vi "RSA306 FFT sweeper2.vi"(0 "Q Array":sgl[](array[numeric]), 1 "2nd Cursor X":dbl, 2 "1st Cursor X":dbl, 3 "Time Array":dbl[](array[numeric]), 5 "1toN Array":i32[](array[numeric]), 7 "I Array":sgl[](array[numeric]), 9 "time step(sec)":dbl, 12 "Freq Center":dbl, 13 "Use windowing":bool, 14 "beta":dbl format="%0.2f") -> (4 "# of Pts Between cursors":dbl, 6 "I & Q  partial":cluster{dbl[], sgl[]}[](graph), 8 "Length out":i32, 10 "FFT^2 from partial":cluster{dbl[], dbl[]}, 15 "FreqStep":dbl)   [LabVIEW 2016]
uses:
  <vilib>/Analysis/4window.llb/Kaiser-Bessel Window (CDB).vi
  <vilib>/Analysis/2dsp.llb/Complex FFT.vi
  <vilib>/Analysis/NI_AALPro.lvlib
panel:
  out "FFT^2  partial":cluster{dbl[], dbl[]}(graph)
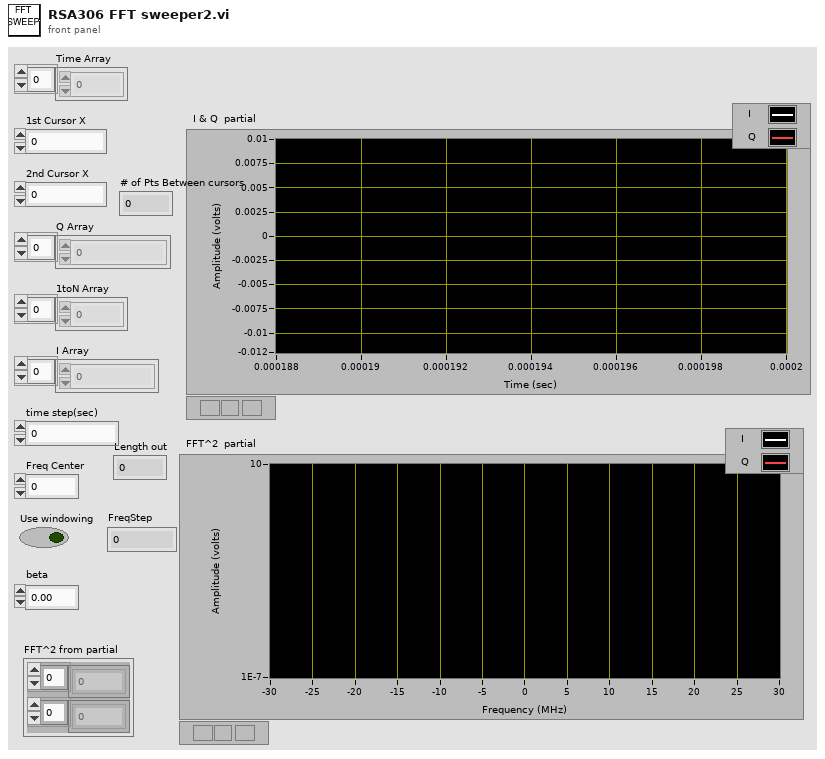
[diagram p1: front panel]
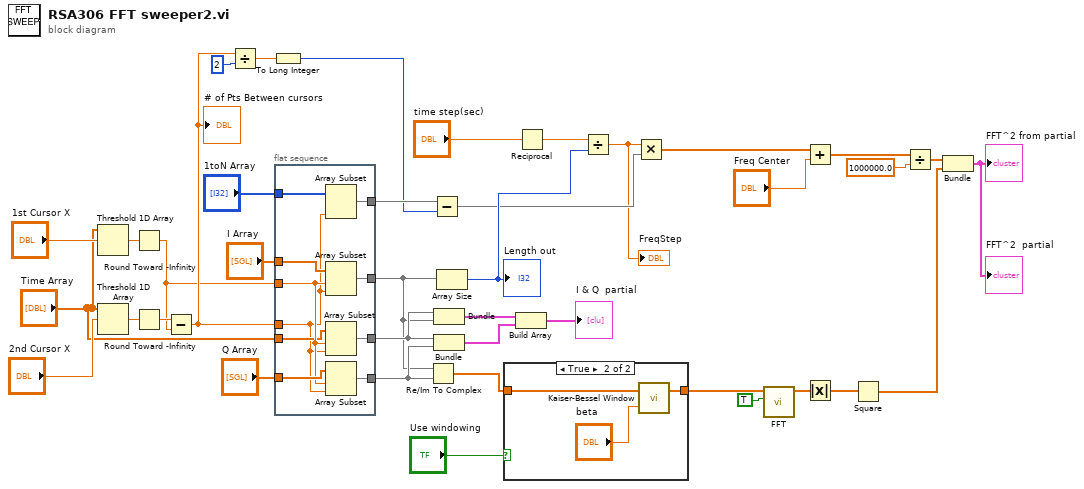
[diagram p0: block diagram]
diagram:
  n1 = Threshold 1D Array(2:"1st Cursor X", 3:"Time Array") -> (0:w24:dbl)  [unwired: 1 in]
  n2 = Threshold 1D Array(2:"2nd Cursor X", 3:"Time Array") -> (0:w25:dbl)  [unwired: 1 in]
  n3 = Round Toward -Infinity(1:w24) -> (0:w26:dbl)
  n4 = Round Toward -Infinity(1:w25) -> (0:w27:dbl)
  n5 = Subtract(x=w27, y=w26) -> (x-y=w35:dbl)
  "# of Pts Between cursors" <- w35
  n6 = Divide(x=w35, y=2) -> (x/y=w32:dbl)
  n7 = To Long Integer(number=w32) -> (32bit integer=w33:i32)
  n8 = flat-sequence {
    tunnel: "I Array" -> [w49]
    tunnel: [w48] -> w13
    tunnel: "Q Array" -> [w47]
    tunnel: [w46] -> w15
    tunnel: w26 -> [w45]
    tunnel: "Time Array" -> [w44]
    tunnel: [w43] -> w29
    tunnel: "1toN Array" -> [w42]
    tunnel: w35 -> [w40]
    tunnel: [w41] -> w36
    frame #0 {
      n9 = Array Subset(array=w42, length=w40) -> (w41:i32[])  [unwired: 1 in]
      n10 = Array Subset(array=w49, index=w45, length=w40) -> (w48:sgl[])
      n11 = Array Subset(array=w44, index=w45, length=w40) -> (w43:dbl[])
      n12 = Array Subset(array=w47, index=w45, length=w40) -> (w46:sgl[])
    }
  }
  n13 = Re/Im To Complex(1:w15, 2:w13) -> (0:w18:csg[])
  n14 = Subtract(x=w36, y=w33) -> (x-y=w9:i32[])
  n15 = Bundle(w29, w13) -> (w5:cluster{dbl[], sgl[]})  [unwired: 1 in]
  n16 = Bundle(w29, w15) -> (w4:cluster{dbl[], sgl[]})  [unwired: 1 in]
  n17 = Array Size(array=w13) -> (size(s)=w37:i32)
  "Length out" <- w37
  n18 = case shown="True" "Use windowing" {
    tunnel: w18 -> [w50 w53]
    tunnel: [w50 w52] -> w30
    frame False {
    }
    frame True {
      n19 = call-poly <vilib>:"Kaiser-Bessel Window.vi"("beta"="beta", "X"=w53) -> ("Windowed X"=w52:cdb[])  [unwired: 1 out]
    }
  }
  n20 = Build Array(w5, w4) -> (→"I & Q  partial":cluster{dbl[], sgl[]}[])
  n21 = Reciprocal(x="time step(sec)") -> (1/x=w1:dbl)
  n22 = Divide(x=w1, y=w37) -> (x/y=w8:dbl)
  "FreqStep" <- w8
  n23 = Multiply(x=w8, y=w9) -> (x*y=w10:dbl[])
  n24 = call-poly <vilib>:"FFT.vi"("shift?"=TRUE, "X"=w30) -> ("FFT {X}"=w11:cdb[])  [unwired: 8 in, 1 out]
  n25 = Add(x=w10, y="Freq Center") -> (x+y=w22:dbl[])
  n26 = Absolute Value(x=w11) -> (abs(x)=w16:dbl[])
  n27 = Square(x=w16) -> (x^2=w17:dbl[])
  n28 = Divide(x=w22, y=1000000.0) -> (x/y=w23:dbl[])
  n29 = Bundle(w23, w17) -> (→"FFT^2 from partial" →"FFT^2  partial":cluster{dbl[], dbl[]})  [unwired: 1 in]
